vi "C2F.vi"(1 "Temperature [C]":dbl) -> (0 "Temperature [F]":dbl)   [LabVIEW 2017]
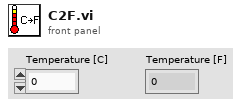
[diagram p1: front panel]
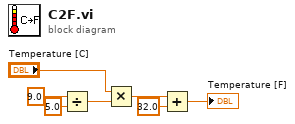
[diagram p0: block diagram]
diagram:
  n1 = Divide(x=9.0, y=5.0) -> (x/y=w4:dbl)
  n2 = Multiply(x="Temperature [C]", y=w4) -> (x*y=w2:dbl)
  n3 = Add(x=w2, y=32.0) -> (x+y=→"Temperature [F]":dbl)
